vi "column BLOB.vi"(8 "error in (no error)":errorcluster, 11 "SQLite3LV Cursor in":refnum<class "cursor.lvclass">) -> (0 "error out":errorcluster, 2 "BLOB":string, 3 "SQLite3LV Cursor out":refnum<class "cursor.lvclass">)   [LabVIEW 2014, in "SQLite3LV.lvlib" / "cursor.lvclass"]
uses:
  cursor.lvclass
  cursor.lvclass/cursor.ctl
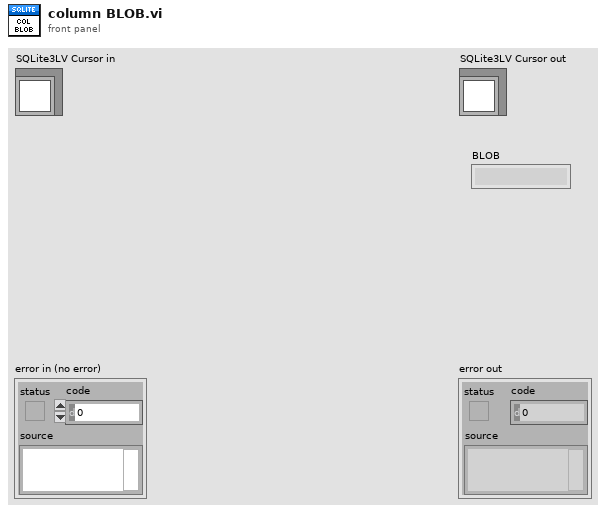
[diagram p1: front panel]
types:
  T1 = typedef "SQLite3LV.lvlib/cursor.lvclass/ctl_active_statement.ctl" = cluster{"ppStmt":i64, "column count":i32, "bind offset":i32, "bind param count":i32, "finished?":bool, "column offset":i32, "column types":i32[]}
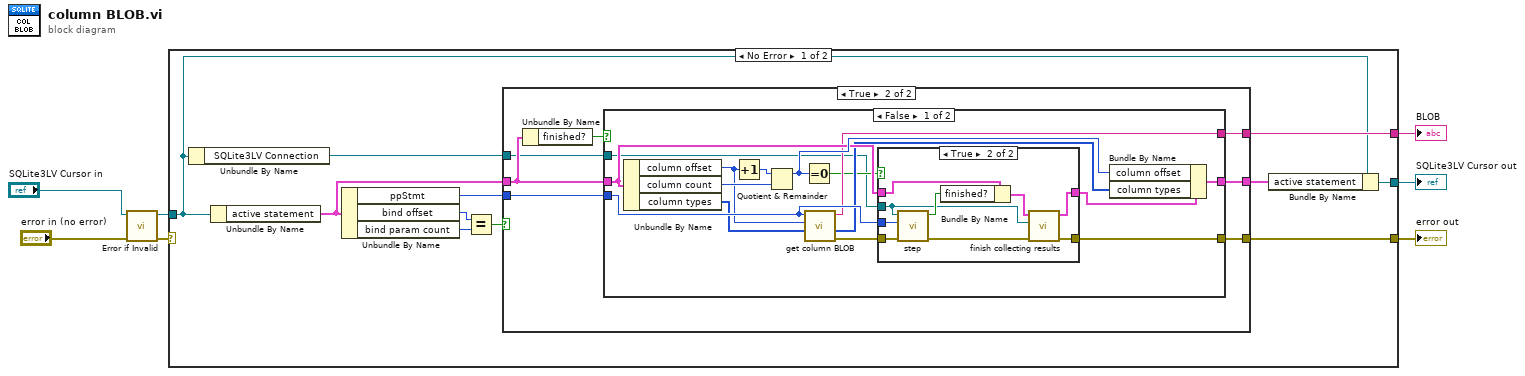
[diagram p0: block diagram]
diagram:
  n1 = call "Error if Invalid.vi"("error in (no error)"="error in (no error)", "SQLite3LV Cursor in"="SQLite3LV Cursor in") -> ("error out"=w3:errorcluster, "SQLite3LV Cursor out"=w1:refnum<class "cursor.lvclass">)  [unwired: 8 in]
  n2 = case shown="No Error" w3 {
    selector: w3 -> [_ w55]
    tunnel: [w10 w55] -> w6
    tunnel: [w16 w54] -> w7
    tunnel: w1 -> [w17 w54]
    tunnel: [w18 _] -> w5
    frame No Error {
      n3 = Unbundle By Name(w17) -> ("SQLite3LV Connection"=w8:refnum<class "sqlite3.lvclass">)
      n4 = Unbundle By Name(w17) -> ("active statement"=w11:T1)
      n5 = Unbundle By Name(w11) -> ("ppStmt"=w13:i64, "bind offset"=w15:i32, "bind param count"=w14:i32)
      n6 = Equal?(x=w15, y=w14) -> (x = y?=w12:bool)
      n7 = case shown="True" w12 {
        tunnel: w13 -> [_ w26]
        tunnel: w11 -> [w19 w25]
        tunnel: [w19 w23] -> w9
        tunnel: [_ w22] -> w10
        tunnel: [_ w21] -> w18
        tunnel: w8 -> [_ w20]
        frame False {
        }
        frame True {
          n8 = Unbundle By Name(w25) -> ("finished?"=w24:bool)
          n9 = case shown="False" w24 {
            tunnel: w26 -> [w40 _]
            tunnel: w25 -> [w34 w53]
            tunnel: [w41 w53] -> w23
            tunnel: [w39 _] -> w22
            tunnel: [w32 _] -> w21
            tunnel: w20 -> [w27 _]
            frame False {
              n10 = Unbundle By Name(w34) -> ("column offset"=w36:i32, "column count"=w38:i32, "column types"=w31:i32[])
              n11 = Increment(x=w36) -> (x+1=w37:i32)
              n12 = Quotient & Remainder(x=w37, y=w38) -> (x-y*floor(x/y)=w35:i32)  [unwired: 1 out]
              n13 = Equal To 0?(x=w35) -> (x = 0?=w28:bool)
              n14 = call "get column BLOB.vi"("column types"=w31, "column index"=w36, "ppStmt"=w40) -> ("error out"=w29:errorcluster, "column types out"=w30:i32[], "BLOB"=w32:string)  [unwired: 6 in]
              n15 = case shown="True" w28 {
                tunnel: w29 -> [w43 w52]
                tunnel: [w43 w51] -> w39
                tunnel: w40 -> [_ w50]
                tunnel: w34 -> [w42 w49]
                tunnel: [w42 w48] -> w33
                tunnel: w27 -> [_ w44]
                frame False {
                }
                frame True {
                  n16 = call "step.vi"("error in (no error)"=w52, "pStmt"=w50, "psqlite"=w44) -> ("error out"=w45:errorcluster, "finished?"=w47:bool)  [unwired: 7 in]
                  n17 = Bundle By Name(cluster=w49, "finished?"=w47) -> (w46:T1)
                  n18 = call "finish collecting results.vi"("error in (no error)"=w45, "psqlite"=w44, "active statement in"=w46) -> ("error out"=w51:errorcluster, "active statement out"=w48:T1)  [unwired: 7 in]
                }
              }
              n19 = Bundle By Name(cluster=w33, "column offset"=w35, "column types"=w30) -> (w41:T1)
            }
            frame True {
            }
          }
        }
      }
      n20 = Bundle By Name(cluster=w17, "active statement"=w9) -> (w16:refnum<class "cursor.lvclass">)
    }
    frame Error {
    }
  }
  "error out" <- w6
  "SQLite3LV Cursor out" <- w7
  "BLOB" <- w5
